vi "Build JSON String.vi"(8 "error in (no error)":errorcluster, 9 "dsf configuration substring":string, 10 "dsf version substring":string, 11 "json version substring":string) -> (0 "error out":errorcluster, 3 "string":string)   [LabVIEW 2017, in "DSF Core.lvlib" / "Configuration Session.lvclass"]
uses:
  Configuration Session.lvclass
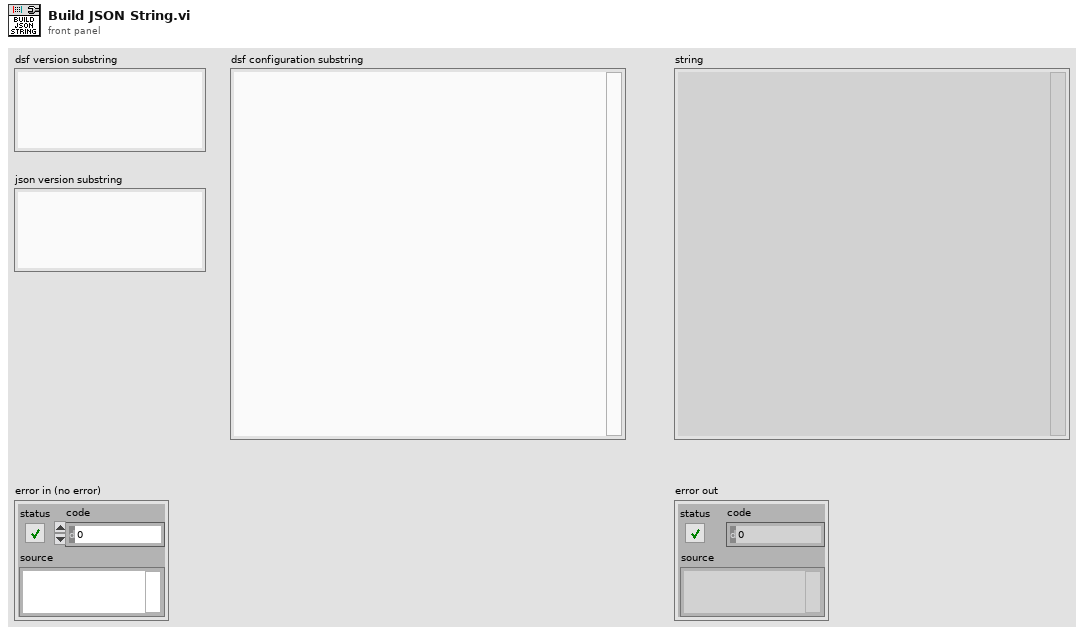
[diagram p1: front panel]
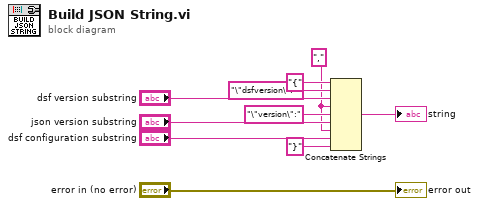
[diagram p0: block diagram]
diagram:
  w3 = "," ("regular expression")
  n1 = Concatenate Strings("{" ("string"), "\"dsfversion\":" ("regular expression"), "dsf version substring", w3, "\"version\":" ("regular expression"), "json version substring", w3, "dsf configuration substring", "}" ("string")) -> (→"string":string)
  "error out" <- "error in (no error)"
